vi "Edgertronic-GetResPlot.vi"(2 "Vertical":dbl=2000.0, 3 "Frame Rate (fps)":dbl, 4 "Horizonal":dbl(slide) scale=0.0..640.0, 5 "picture":picture) -> (0 "Vertical":dbl(slide) scale=0.0..512.0, 1 "2D Picture":picture)   [LabVIEW 2015]
panel:
  in  "Image Size":cluster{"Hmax":dbl, "Vmax":dbl}={"Hmax"=1280.0, "Vmax"=1024.0}
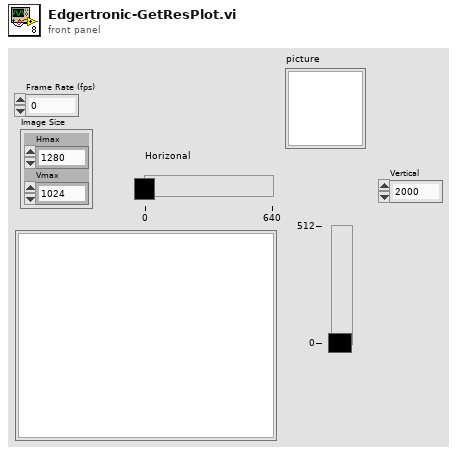
[diagram p1: front panel]
types:
  T1 = cluster{"Width":u16, "Style":enum32{"Solid", "Dash", "Dot", "DashDot", "DashDotDot"}}
  T2 = cluster{"left":i16, "top":i16, "right":i16, "bottom":i16}
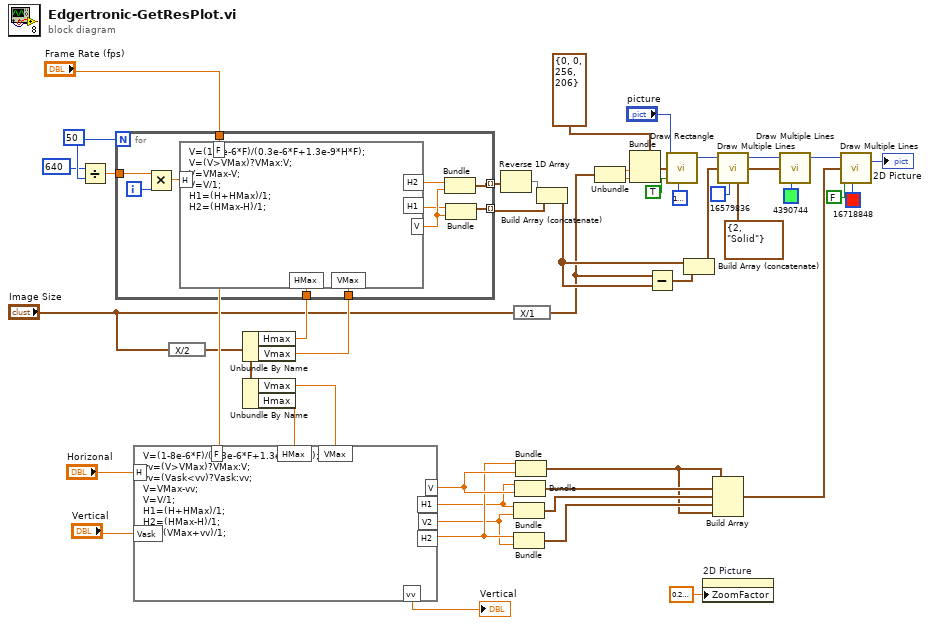
[diagram p0: block diagram]
diagram:
  w38 = 50
  n1 = Divide(x=640, y=w38) -> (x/y=w39:dbl)
  n2 = expression code="X/2"("Image Size") -> (w10:cluster{"Hmax":dbl, "Vmax":dbl})
  n3 = Unbundle By Name(w10) -> ("Hmax"=w15:dbl, "Vmax"=w14:dbl)
  n4 = for {
    N: w38 -> [_]
    tunnel: w39 -> [w57]
    tunnel: "Frame Rate (fps)" -> [w55]
    tunnel: [w54] -> w27 mode=indexing
    tunnel: [w51] -> w26 mode=indexing
    tunnel: w15 -> [w48]
    tunnel: w14 -> [w47]
    i -> [w56]
    n5 = Multiply(x=w57, y=w56) -> (x*y=w53:dbl)
    n6 = formula code="V=(1-8e-6*F)/(0.3e-6*F+1.3e-9*H*F);\nV=(V>VMax)?VMax:V;\nV=VMax-V;\nV=V/1;\nH1=(H+HMax)/1;\nH2=(HMax-H)/1;"("H"=w53, "F"=w55, "HMax"=w48, "VMax"=w47) -> ("V"=w52:dbl, "H1"=w50:dbl, "H2"=w49:dbl)
    n7 = Bundle("H2"=w49, "V"=w52) -> (w51:cluster{"H2":dbl, "V":dbl})  [unwired: 1 in]
    n8 = Bundle("H1"=w50, "V"=w52) -> (w54:cluster{"H1":dbl, "V":dbl})  [unwired: 1 in]
  }
  n9 = Unbundle By Name(w10) -> ("Vmax"=w12:dbl, "Hmax"=w13:dbl)
  n10 = formula code="V=(1-8e-6*F)/(0.3e-6*F+1.3e-9*H*F);\nvv=(V>VMax)?VMax:V;\nvv=(Vask<vv)?Vask:vv;\nV=VMax-vv;\nV=V/1;\nH1=(H+HMax)/1;\nH2=(HMax-H)/1;\nV2=(VMax+vv)/1;"("H"="Horizonal", "F"="Frame Rate (fps)", "HMax"=w13, "VMax"=w12, "Vask"="Vertical") -> ("V"=w20:dbl, "vv"=→"Vertical":dbl, "H2"=w18:dbl, "H1"=w17:dbl, "V2"=w16:dbl)
  n11 = Reverse 1D Array(array=w26) -> (reversed array=w25:cluster{"H2":dbl, "V":dbl}[])
  n12 = expression code="X/1"("Image Size") -> (w8:cluster{"Hmax":dbl, "Vmax":dbl})
  n13 = Bundle("H1"=w17, "V2"=w16) -> (w41:cluster{"H1":dbl, "V2":dbl})  [unwired: 1 in]
  n14 = Bundle("H2"=w18, "V2"=w16) -> (w33:cluster{"H2":dbl, "V2":dbl})  [unwired: 1 in]
  n15 = Bundle("H1"=w17, "V"=w20) -> (w42:cluster{"H1":dbl, "V":dbl})  [unwired: 1 in]
  n16 = Bundle("H2"=w18, "V"=w20) -> (w19:cluster{"H2":dbl, "V":dbl})  [unwired: 1 in]
  n17 = Build Array (concatenate)(w25, w27) -> (w24:cluster{"H1":dbl, "V":dbl}[])
  n18 = Unbundle(w8) -> ("Hmax"=w7:dbl, "Vmax"=w6:dbl)
  n19 = Bundle(cluster=T2 {"left"=0, "top"=0, "right"=256, "bottom"=206} ("rect"), "right"=w7, "bottom"=w6) -> (w5:T2)  [unwired: 2 in]
  n20 = Subtract(x=w8, y=w24) -> (x-y=w23:cluster{dbl, dbl}[])
  n21 = call <vilib>:"Draw Rectangle.vi"("picture"="picture", "rect"=w5, "fill?(F)"=TRUE, "color(black)"=u32 16777216) -> ("new picture"=w32:picture)  [unwired: 5 in]
  n22 = Build Array (concatenate)(w24, w23) -> (w22:cluster{"H1":dbl, "V":dbl}[])
  n23 = property on="2D Picture" class="Pict"("ZoomFactor"=sgl 0.2 ("Zoom Factor")) -> ()  [unwired: 2 in, 2 out]
  n24 = Build Array(w19, w42, w41, w33, w19) -> (w43:cluster{"H2":dbl, "V":dbl}[])
  n25 = call <vilib>:"Draw Multiple Lines.vi"("picture"=w32, "line endpoints"=w22, "color(black)"=u32 16579836, "pen"=T1 {"Width"=2, "Style"=enum."Solid"}) -> ("new picture"=w31:picture)  [unwired: 5 in]
  n26 = call <vilib>:"Draw Multiple Lines.vi"("picture"=w31, "line endpoints"=w22, "color(black)"=u32 4390744) -> ("new picture"=w44:picture)  [unwired: 6 in]
  n27 = call <vilib>:"Draw Multiple Lines.vi"("picture"=w44, "line endpoints"=w43, "fill?(F)"=FALSE, "color(black)"=u32 16718848) -> ("new picture"=→"2D Picture":picture)  [unwired: 5 in]
